vi "FA_GetFIRSTdata.vi"(8 "Error In":errorcluster) -> (0 "Error Out":errorcluster)   [LabVIEW 2013, in "FA_FIRST.lvlib"]
uses:
  FA_FIRST.lvlib
  FIRST Client/source/VI Source/FC_Competition Attributes.ctl
  FIRST Client/source/VI Source/FC_Team Attributes.ctl
  FIRST Client/source/VI Source/FC_Target.ctl
  FA_LocalStore API/source/VI Source/FA_LSSpecialTypes.ctl
  FIRST Client/source/VI Source/FC_FIRST Client.lvlib
  FA_LocalStore API/source/VI Source/FA_LocalStore.lvlib
panel:
  out "Attendance Debug":string[][](array[string])
  out "Team Info Debug":T1[](array[typedef])
  out "Event Info Debug":T2[](array[typedef])
  # "Team Numbers attending each event (from Event Info)"
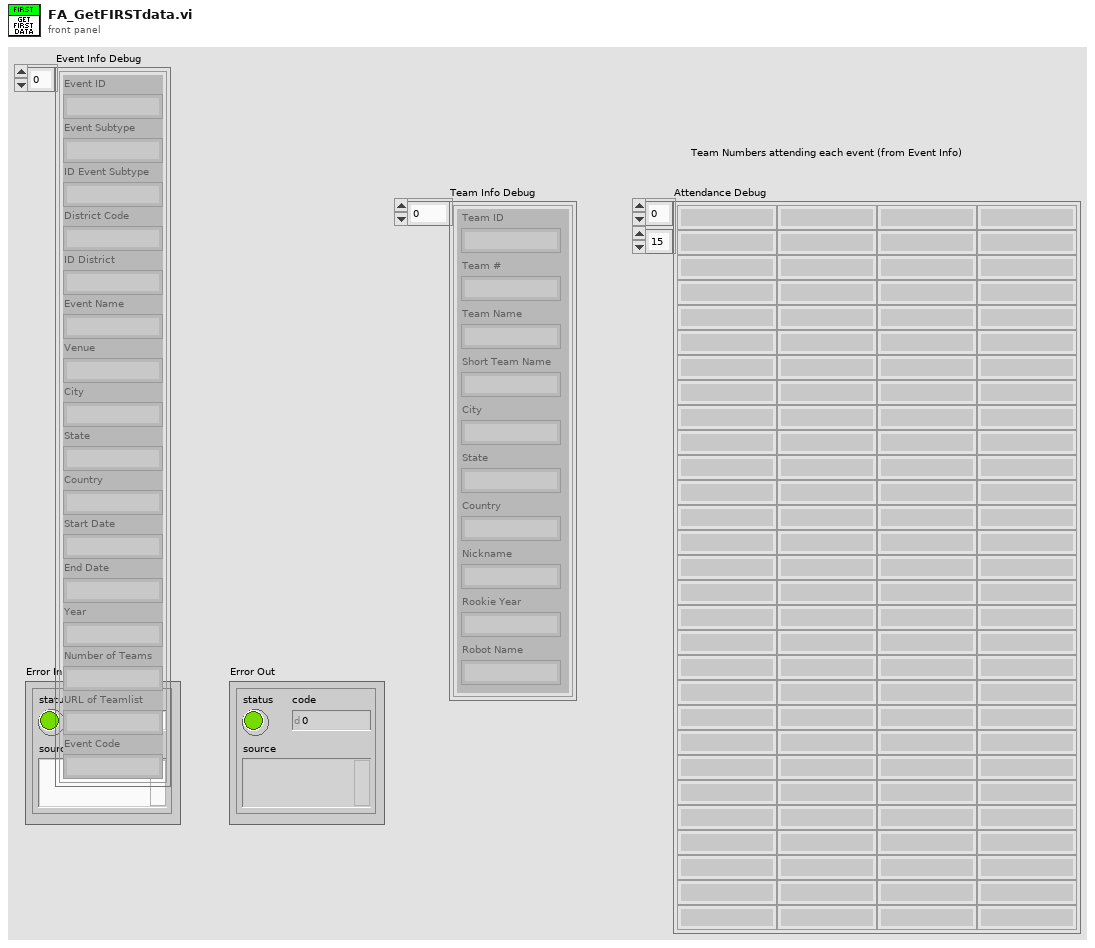
[diagram p1: front panel]
types:
  T1 = typedef "FC_FIRST Client.lvlib/FC_Team Attributes.ctl" = cluster{"Team ID":string, "Team #":string, "Team Name":string, "Short Team Name":string, "City":string, "State":string, "Country":string, "Nickname":string, "Rookie Year":string, "Robot Name":string}
  T2 = typedef "FC_FIRST Client.lvlib/FC_Competition Attributes.ctl" = cluster{"Event ID":string, "Event Subtype":string, "ID Event Subtype":string, "District Code":string, "ID District":string, "Event Name":string, "Venue":string, "City":string, "State":string, "Country":string, "Start Date":string, "End Date":string, "Year":string, "Number of Teams":string, "URL of Teamlist":string, "Event Code":string}
  T3 = typedef "FA_LocalStore.lvlib/FA_LSSpecialTypes.ctl" = string
  T4 = typedef "FC_FIRST Client.lvlib/FC_Target.ctl" = enum16{"Teams", "Competitions"}
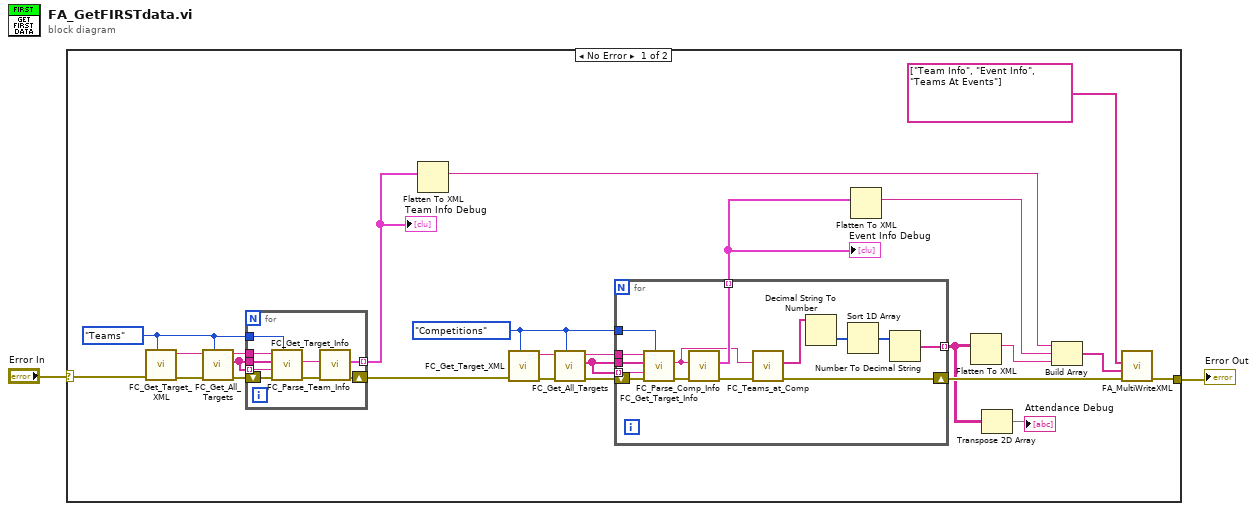
[diagram p0: block diagram]
diagram:
  n1 = case shown="No Error" "Error In" {
    selector: "Error In" -> [w12 w51]
    tunnel: [w19 w51] -> w1
    frame No Error {
      w14 = FC_Target."Teams" ("Enum")
      w23 = FC_Target."Competitions" ("Target")
      n2 = call "FC_Get_Target_XML.vi"("Target"=w14, "error in"=w12) -> ("error out"=w15:errorcluster, "All Teams XML"=w18:string)  [unwired: 8 in]
      n3 = call "FC_Get_All_Targets.vi"("Target"=w14, "Error In"=w15, "Target XML"=w18) -> ("error out"=w16:errorcluster, "Array of Targets"=w13:string[], "Copy of Target XML"=w17:string)  [unwired: 6 in]
      n4 = for {
        tunnel: w17 -> [w36]
        tunnel: w14 -> [w34]
        tunnel: w13 -> [w33]
        tunnel: w13 -> [w30] mode=indexing
        shift-right: [w29] -> w4
        shift-left: w16 -> [w35]
        tunnel: [w28] -> w10 mode=indexing
        n5 = call "FC_Get_Target_Info.vi"("Target"=w34, "Error In"=w35, "Desired Target"=w30, "Array of Targets"=w33, "Target XML"=w36) -> ("error out"=w31:errorcluster, "Target Info"=w32:string)  [unwired: 5 in]
        n6 = call "FC_Parse_Team_Info.vi"("Error In"=w31, "All Team Data"=w32) -> ("Error Out"=w29:errorcluster, "Team Data Cluster"=w28:T1)  [unwired: 8 in]
      }
      "Team Info Debug" <- w10
      n7 = Flatten To XML(anything=w10) -> (xml string=w7:string)
      n8 = call "FC_Get_Target_XML.vi"("Target"=w23, "error in"=w4) -> ("error out"=w27:errorcluster, "All Teams XML"=w26:string)  [unwired: 8 in]
      n9 = call "FC_Get_All_Targets.vi"("Target"=w23, "Error In"=w27, "Target XML"=w26) -> ("error out"=w25:errorcluster, "Array of Targets"=w22:string[], "Copy of Target XML"=w24:string)  [unwired: 6 in]
      n10 = for {
        tunnel: w24 -> [w49]
        tunnel: w23 -> [w48]
        tunnel: w22 -> [w47]
        tunnel: w22 -> [w46] mode=indexing
        tunnel: [w42] -> w21 mode=indexing
        shift-right: [w44] -> w11
        shift-left: w25 -> [w50]
        tunnel: [w37] -> w5 mode=indexing
        n11 = call "FC_Get_Target_Info.vi"("Target"=w48, "Error In"=w50, "Desired Target"=w46, "Array of Targets"=w47, "Target XML"=w49) -> ("error out"=w43:errorcluster, "Target Info"=w41:string)  [unwired: 5 in]
        n12 = call "FC_Parse_Comp_Info.vi"("Error In"=w43, "All Competition Data"=w41) -> ("Error Out"=w45:errorcluster, "Comp Data Cluster"=w42:T2)  [unwired: 8 in]
        n13 = call "FC_Teams_at_Comp.vi"("error constant"=w45, "Event ID"=w41) -> ("error out"=w44:errorcluster, "Array of Team Numbers"=w38:string[])  [unwired: 8 in]
        n14 = Decimal String To Number(string=w38) -> (number=w39:i32[])  [unwired: 2 in, 1 out]
        n15 = Sort 1D Array(array=w39) -> (sorted array=w40:i32[])
        n16 = Number To Decimal String(number=w40) -> (decimal integer string=w37:string[])  [unwired: 1 in]
      }
      "Event Info Debug" <- w21
      n17 = Flatten To XML(anything=w21) -> (xml string=w8:string)
      n18 = Flatten To XML(anything=w5) -> (xml string=w9:string)
      n19 = Transpose 2D Array(2D array=w5) -> (transposed array=→"Attendance Debug":string[][])
      n20 = Build Array(w7, w8, w9) -> (w6:string[])
      n21 = call "FA_MultiWriteXML.vi"("Error In"=w11, "XML String Array"=w6, "Special Type Array"=T3[] ["Team Info", "Event Info", "Teams At Events"]) -> ("Error Out"=w19:errorcluster)  [unwired: 6 in]
    }
    frame Error {
    }
  }
  "Error Out" <- w1
